vi "Calculate Focal Lengths in Pixels.vi"(9 "Robot Calibration Cluster":T1={"Camera Height on robot (in)"=34.5, "Camera Angle on the robot (deg)"=28.3, "Camera FOV Vert View Angle (deg)"=0.946, "Camera FOV Hor View Angle (deg)"=26.5, "Camera Focal Length (mm)"=10.0, "Target size (in)"=6.5} {"Camera FOV Hor View Angle (deg)" format="%#_13g"; "Camera Focal Length (mm)" format="%#_13g"; "Target size (in)" format="%#_13g"; "Camera FOV Vert View Angle (deg)" format="%#_13g"; "Camera Angle on the robot (deg)" format="%#_13g"; "Camera Height on robot (in)" format="%#_13g"}, 10 "Picture Cluster":cluster{"X Resolution":i32, "Y Resolution":i32}) -> (1 "fy":dbl, 2 "fx":dbl)   [LabVIEW 2025]
uses:
  Camera Info.ctl
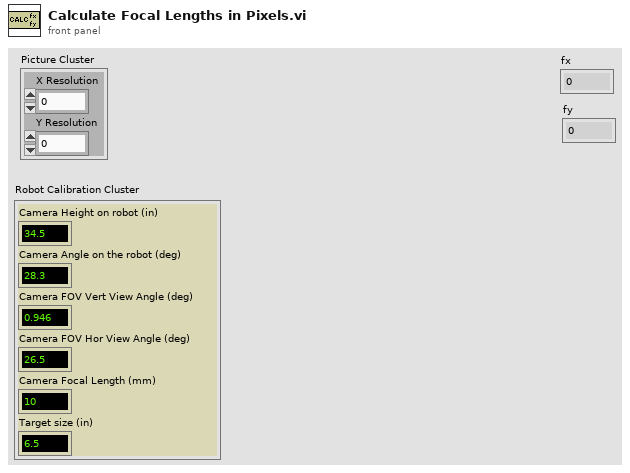
[diagram p1: front panel]
types:
  T1 = typedef "Camera Info.ctl" = cluster{"Camera Height on robot (in)":dbl, "Camera Angle on the robot (deg)":dbl, "Camera FOV Vert View Angle (deg)":dbl, "Camera FOV Hor View Angle (deg)":dbl, "Camera Focal Length (mm)":dbl, "Target size (in)":dbl}
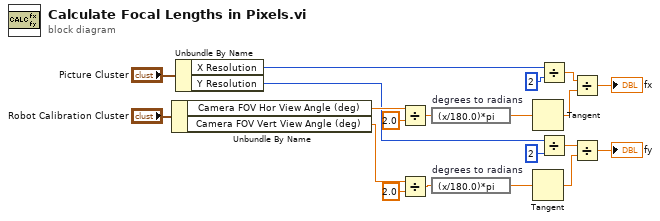
[diagram p0: block diagram]
diagram:
  n1 = Unbundle By Name("Robot Calibration Cluster") -> ("Camera FOV Hor View Angle (deg)"=w16:dbl, "Camera FOV Vert View Angle (deg)"=w2:dbl)
  n2 = Unbundle By Name("Picture Cluster") -> ("X Resolution"=w18:i32, "Y Resolution"=w9:i32)
  n3 = Divide(x=w16, y=2.0) -> (x/y=w12:dbl)
  n4 = Divide(x=w2, y=2.0) -> (x/y=w1:dbl)
  n5 = expression code="(x/180.0)*pi" "degrees to radians"(w12) -> (w11:dbl)
  n6 = expression code="(x/180.0)*pi" "degrees to radians"(w1) -> (w8:dbl)
  n7 = Tangent(1:w11) -> (0:w13:dbl)
  n8 = Tangent(1:w8) -> (0:w6:dbl)
  n9 = Divide(x=w18, y=2) -> (x/y=w14:dbl)
  n10 = Divide(x=w9, y=2) -> (x/y=w7:dbl)
  n11 = Divide(x=w14, y=w13) -> (x/y=→"fx":dbl)
  n12 = Divide(x=w7, y=w6) -> (x/y=→"fy":dbl)
